vi "NaN_screening.vi"(11 "Input":T1 {"File Location" items=["Unknown"=-5, "IDL Processing"=-4, "Writing from Queue"=-3, "Labview Files"=-2, "Retry Labview files"=-1, "Local Cache "=0, "Storage"=1]}) -> (3 "Output":T1 {"File Location" items=["Unknown"=-5, "IDL Processing"=-4, "Writing from Queue"=-3, "Labview Files"=-2, "Retry Labview files"=-1, "Local Cache "=0, "Storage"=1]})   [LabVIEW 2013]
uses:
  Public API/Post_Dust_Event.ctl
  Controls/File_location.ctl
panel:
  # "Dust Event"
  # "Dust Event"
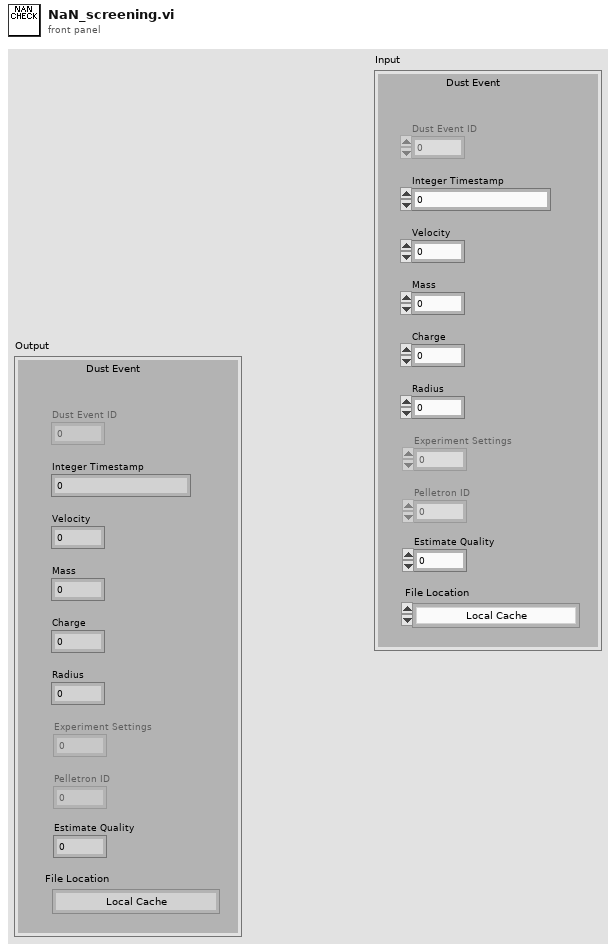
[diagram p1: front panel]
types:
  T1 = typedef "Post_Dust_Event.ctl" = cluster{"Dust Event ID":i64, "Integer Timestamp":i64, "Velocity":sgl, "Mass":sgl, "Charge":sgl, "Radius":sgl, "Experiment Settings":dbl, "Pelletron ID":i32, "Estimate Quality":sgl, "File Location":T2, "id_dust_info":dbl}
  T2 = typedef "File_location.ctl" = i8
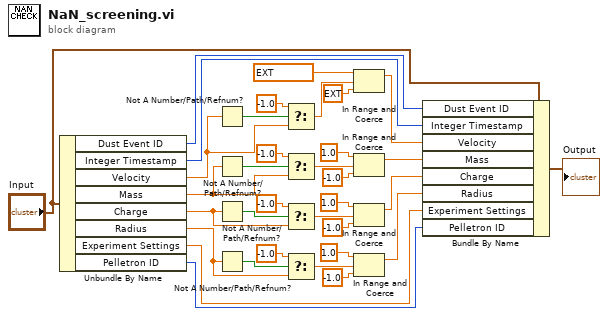
[diagram p0: block diagram]
diagram:
  n1 = Unbundle By Name("Input") -> ("Dust Event ID"=w32:i64, "Integer Timestamp"=w31:i64, "Velocity"=w19:sgl, "Mass"=w21:sgl, "Charge"=w23:sgl, "Radius"=w18:sgl, "Experiment Settings"=w30:dbl, "Pelletron ID"=w29:i32)
  n2 = Not A Number/Path/Refnum?(number/path/refnum=w19) -> (NaN/Path/Refnum?=w20:bool)
  n3 = Not A Number/Path/Refnum?(number/path/refnum=w21) -> (NaN/Path/Refnum?=w22:bool)
  n4 = Not A Number/Path/Refnum?(number/path/refnum=w23) -> (NaN/Path/Refnum?=w25:bool)
  n5 = Not A Number/Path/Refnum?(number/path/refnum=w18) -> (NaN/Path/Refnum?=w17:bool)
  n6 = Select(t=-1.0 ("y"), s=w20, f=w19) -> (s? t:f=w14:dbl)
  n7 = Select(t=-1.0 ("y"), s=w22, f=w21) -> (s? t:f=w10:dbl)
  n8 = Select(t=-1.0 ("y"), s=w25, f=w23) -> (s? t:f=w4:dbl)
  n9 = Select(t=-1.0 ("y"), s=w17, f=w18) -> (s? t:f=w2:dbl)
  n10 = In Range and Coerce(upper limit=ext 299792458.0, x=w14, lower limit=ext -1.0) -> (coerced(x)=w13:ext)  [unwired: 1 out]
  n11 = In Range and Coerce(upper limit=1.0, x=w10, lower limit=-1.0) -> (coerced(x)=w9:dbl)  [unwired: 1 out]
  n12 = In Range and Coerce(upper limit=1.0, x=w4, lower limit=-1.0) -> (coerced(x)=w3:dbl)  [unwired: 1 out]
  n13 = In Range and Coerce(upper limit=1.0, x=w2, lower limit=-1.0) -> (coerced(x)=w1:dbl)  [unwired: 1 out]
  n14 = Bundle By Name(cluster="Input", "Dust Event ID"=w32, "Integer Timestamp"=w31, "Velocity"=w13, "Mass"=w9, "Charge"=w3, "Radius"=w1, "Experiment Settings"=w30, "Pelletron ID"=w29) -> (→"Output":T1)
